vi "Comments.Add Wiring Description.vi"(8 "error in (no error)":errorcluster, 11 "Control Experiment":refnum<class "SMO.Control Experiment.lvclass">) -> (0 "error out":errorcluster, 2 "Wiring Description":string, 3 "Control Experiment out":refnum<class "SMO.Control Experiment.lvclass">)   [LabVIEW 2019, in "SMO.Control Experiment.lvclass"]
uses:
  SMO.Control Experiment.lvclass
  <userlib>/LevyLab/PLYM/YAML.lvclass
  <userlib>/LevyLab/Krohn Hite 7008/Instrument.KH7008.lvclass
panel:
  out "Numeric":i32
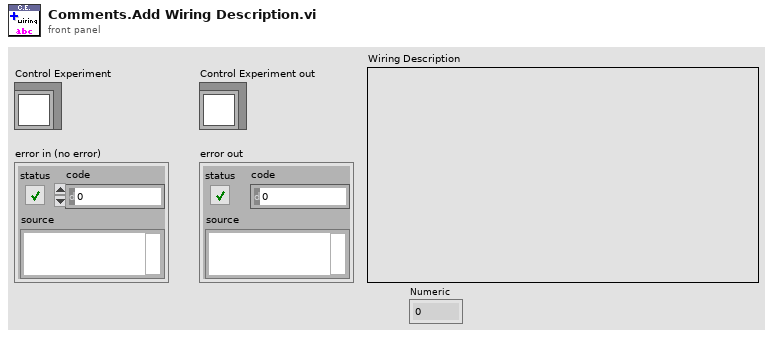
[diagram p1: front panel]
types:
  T1 = typedef "SMO.Control Experiment.lvclass/Wiring Description--cluster.ctl" = cluster{"AI":cluster{"Channel":u32, "Gain":dbl}, "Device":cluster{"Electrode":string, "Label":string, "Type":string}, "KH":cluster{"Channel":string, "Configuration":string, "Gain":u32, "Shunt Resistor":u32}, "AO":cluster{"Channel":u32, "Gain":dbl}}[]
  T2 = typedef "Instrument.KH7008.lvclass/SetAll-Array.ctl" = T3[]
  T3 = typedef "Instrument.KH7008.lvclass/SetAll-Cluster.ctl" = cluster{"Channel":T4, "Gain":T5, "Bandwidth Filter":T6, "Shunt Resistor":T7, "Coupling":T8, "Input Config":T9}
  T4 = typedef "Instrument.KH7008.lvclass/Channel-Enum.ctl" = enum16{"Channel 1", "Channel 2", "Channel 3", "Channel 4", "Channel 5", "Channel 6", "Channel 7", "Channel 8"}
  T5 = typedef "Instrument.KH7008.lvclass/Gain-Enum.ctl" = enum16{"1x", "10x", "100x", "1000x"}
  T6 = typedef "Instrument.KH7008.lvclass/Filter-Enum.ctl" = enum16{"OFF", "ON"}
  T7 = typedef "Instrument.KH7008.lvclass/Shunt-Enum.ctl" = enum16{"Open", "50 Ohms", "500 Ohms", "5k Ohms", "50k Ohms", "10M Ohm"}
  T8 = typedef "Instrument.KH7008.lvclass/Coupling-Enum.ctl" = enum16{"AC", "DC"}
  T9 = typedef "Instrument.KH7008.lvclass/Input Configuration-Enum.ctl" = enum16{"Ground", "SE+ (-gnd)", "SE- (+gnd)", "Differential"}
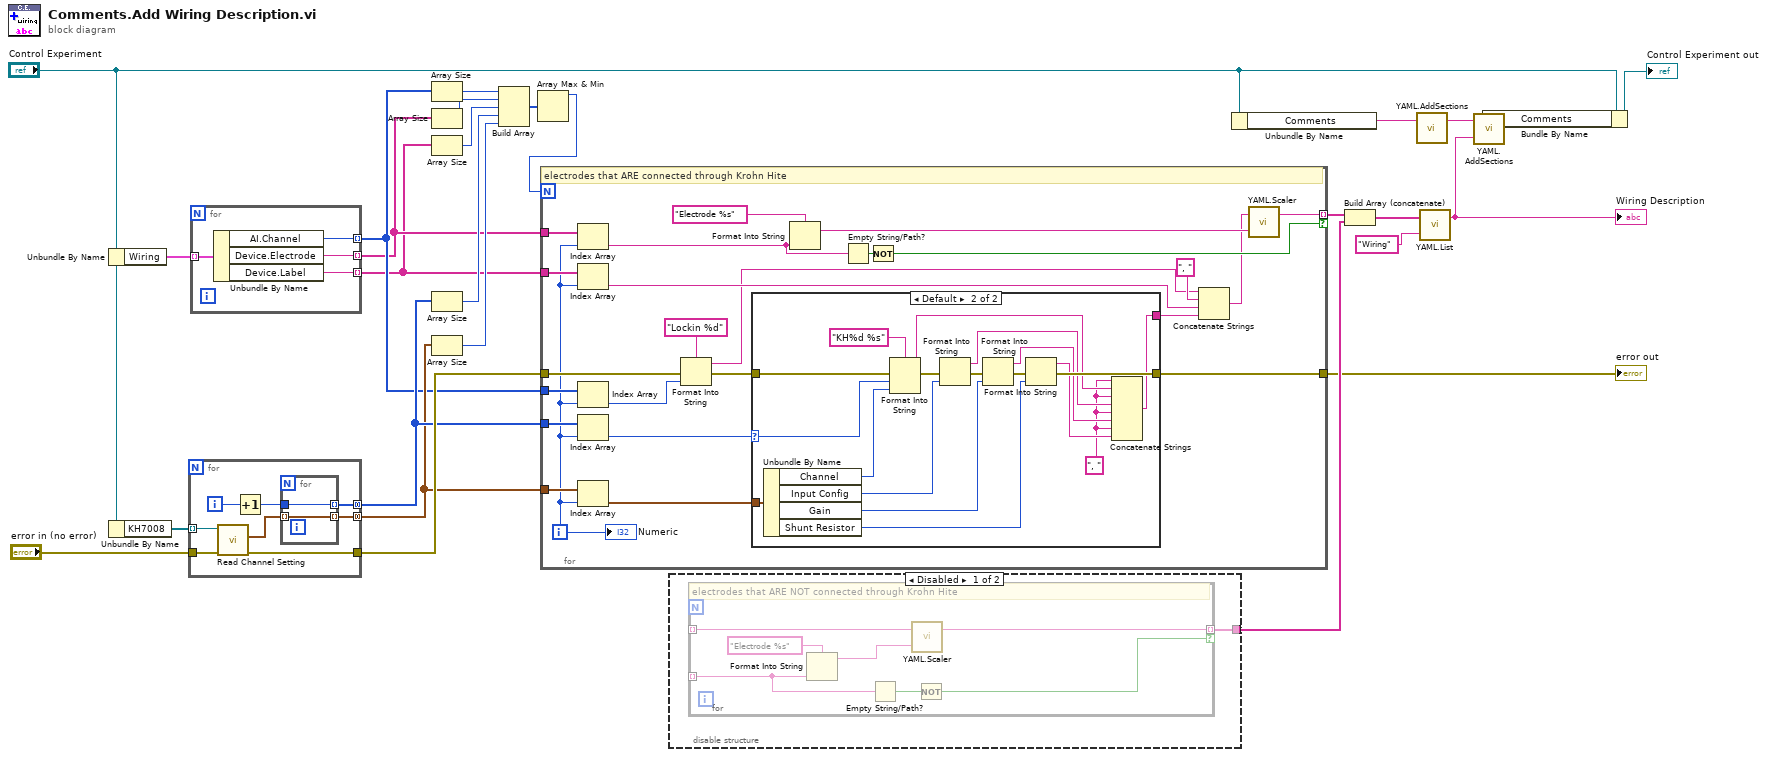
[diagram p0: block diagram]
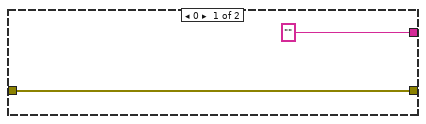
[diagram p3: hidden frame]
diagram:
  n1 = Unbundle By Name("Control Experiment") -> ("Wiring"=w4:T1)
  n2 = Unbundle By Name("Control Experiment") -> ("KH7008"=w18:refnum<class "Instrument.KH7008.lvclass">[])
  n3 = for {
    tunnel: [w29] -> w13 mode=concatenating
    tunnel: w18 -> [w34] mode=indexing
    tunnel: "error in (no error)" -> [w33]
    tunnel: [w35] -> w19
    tunnel: [w28] -> w14 mode=concatenating
    i -> [w32]
    n4 = call <userlib>:"Read Channel Setting.vi"("error in (no error)"=w33, "Instrument.KH7008 in"=w34) -> ("error out"=w35:errorcluster, "Channel Setting"=w30:T2)  [unwired: 7 in, 1 out]
    n5 = Increment(x=w32) -> (x+1=w31:i32)
    n6 = for {
      tunnel: w31 -> [w37]
      tunnel: w30 -> [w36] mode=indexing
      tunnel: [w37] -> w28 mode=indexing
      tunnel: [w36] -> w29 mode=indexing
    }
  }
  n7 = for {
    tunnel: w4 -> [w41] mode=indexing
    tunnel: [w40] -> w3 mode=indexing
    tunnel: [w39] -> w2 mode=indexing
    tunnel: [w38] -> w1 mode=indexing
    n8 = Unbundle By Name(w41) -> ("AI.Channel"=w40:u32, "Device.Electrode"=w39:string, "Device.Label"=w38:string)
  }
  n9 = Array Size(array=w3) -> (size(s)=w12:i32)
  n10 = Array Size(array=w2) -> (size(s)=w11:i32)
  n11 = Array Size(array=w1) -> (size(s)=w10:i32)
  n12 = Array Size(array=w14) -> (size(s)=w9:i32)
  n13 = Array Size(array=w13) -> (size(s)=w8:i32)
  n14 = Build Array(w12, w11, w10, w9, w8) -> (w7:i32[])
  n15 = Array Max & Min(array=w7) -> (max value=w6:i32)  [unwired: 3 out]
  n16 = for {
    N: w6 -> [_]
    tunnel: w3 -> [w53]
    tunnel: w2 -> [w60]
    tunnel: w1 -> [w52]
    tunnel: [w57] -> w21 mode=indexing if=w63
    tunnel: w19 -> [w59]
    tunnel: [w55] -> w17
    tunnel: w13 -> [w62]
    tunnel: w14 -> [w54]
    i -> [w42]
    # "electrodes that ARE connected through Krohn Hite"
    n17 = Index Array(array=w60, index=w42) -> (element=w50:string)
    n18 = Index Array(array=w52, index=w42) -> (element=w44:string)
    n19 = Index Array(array=w53, index=w42) -> (element=w51:u32)
    n20 = Index Array(array=w54, index=w42) -> (element=w46:i32)
    n21 = Index Array(array=w62, index=w42) -> (element=w49:T3)
    n22 = Format Into String(format string="Lockin %d", error in=w59, w51) -> (resulting string=w43:string, error out=w65:errorcluster)  [unwired: 1 in]
    n23 = case shown="Default" w46 {
      selector: w46 -> [_ w68]
      tunnel: w65 -> [w67 w82]
      tunnel: ["" w69] -> w45
      tunnel: [w67 w76] -> w55
      tunnel: w49 -> [_ w75]
      frame 0 {
      }
      frame Default {
        w70 = ", "
        n24 = Unbundle By Name(w75) -> ("Channel"=w77:T4, "Input Config"=w81:T9, "Gain"=w80:T5, "Shunt Resistor"=w79:T7)
        n25 = Format Into String(format string="KH%d %s", error in=w82, w68, w77) -> (resulting string=w71:string, error out=w85:errorcluster)  [unwired: 1 in]
        n26 = Format Into String(error in=w85, w81) -> (resulting string=w72:string, error out=w84:errorcluster)  [unwired: 2 in]
        n27 = Format Into String(error in=w84, w80) -> (resulting string=w73:string, error out=w83:errorcluster)  [unwired: 2 in]
        n28 = Format Into String(error in=w83, w79) -> (resulting string=w74:string, error out=w76:errorcluster)  [unwired: 2 in]
        n29 = Concatenate Strings(w70, w71, w70, w72, w70, w73, w70, w74) -> (w69:string)
      }
    }
    n30 = Format Into String(format string="Electrode %s", w50) -> (resulting string=w58:string)  [unwired: 2 in, 1 out]
    n31 = Empty String/Path?(string/path=w50) -> (empty?=w64:bool)
    n32 = Not(x=w64) -> (.not. x?=w63:bool)
    n33 = Concatenate Strings(w43, ", ", w44, w45) -> (w48:string)
    n34 = call <userlib>:"YAML.Scaler.vi"("Key"=w58, "Scaler"=w48) -> ("Output"=w57:string)  [unwired: 1 in]
    "Numeric" <- w42
  }
  "error out" <- w17
  n35 = disable-structure shown="Disabled" {
    disable-tunnel: [w86 _] -> w22
    frame Disabled {
      n36 = for {
        tunnel: [w87] -> w86 mode=indexing if=w91
        tunnel: _ -> [w88] mode=indexing
        tunnel: _ -> [w93] mode=indexing
        # "electrodes that ARE NOT connected through Krohn Hite"
        n37 = Format Into String(format string="Electrode %s", w93) -> (resulting string=w89:string)  [unwired: 2 in, 1 out]
        n38 = Empty String/Path?(string/path=w93) -> (empty?=w92:bool)
        n39 = call <userlib>:"YAML.Scaler.vi"("Key"=w89, "Scaler"=w88) -> ("Output"=w87:string)  [unwired: 1 in]
        n40 = Not(x=w92) -> (.not. x?=w91:bool)
      }
    }
    frame Enabled {
    }
  }
  n41 = Unbundle By Name("Control Experiment") -> ("Comments"=w24:string)
  n42 = Build Array (concatenate)(w21, w22) -> (w23:string[])
  n43 = call <userlib>:"YAML.AddSections.vi"("Section 1"=w24) -> ("Output"=w26:string)  [unwired: 2 in]
  n44 = call <userlib>:"YAML.List.vi"("Key"="Wiring" ("string"), "lines"=w23) -> ("Output"=w15:string)  [unwired: 1 in]
  "Wiring Description" <- w15
  n45 = call <userlib>:"YAML.AddSections.vi"("Section 2"=w15, "Section 1"=w26) -> ("Output"=w27:string)  [unwired: 1 in]
  n46 = Bundle By Name(cluster="Control Experiment", "Comments"=w27) -> (→"Control Experiment out":refnum<class "SMO.Control Experiment.lvclass">)
